vi "Byte Array.vi"(8 "Error In":errorcluster) -> (0 "Error Out":errorcluster)   [LabVIEW 2017, in "Tests.lvlib" / "To Msgpack.lvlib"]
uses:
  To Msgpack.lvlib
  <vilib>/addons/_JKI Toolkits/Caraya/classes/Test/Test.lvclass
  src/LabPack/LabPack.lvlib
  <vilib>/addons/_JKI Toolkits/Caraya/classes/Assert/Assert.lvclass
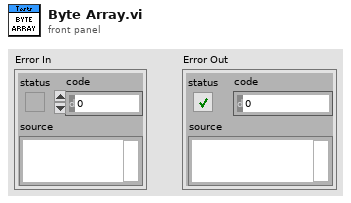
[diagram p1: front panel]
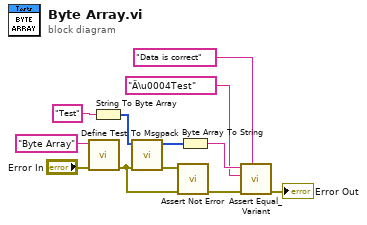
[diagram p0: block diagram]
diagram:
  n1 = call <vilib>:"Define Test.vi"("error in (no error)"="Error In", "Label (VI Title)"="Byte Array") -> ("error out"=w8:errorcluster)  [unwired: 9 in]
  n2 = String To Byte Array(string="Test") -> (unsigned byte array=w1:u8[])
  n3 = call "To Msgpack.vi"("Error In"=w8, "Anything"=w1) -> ("Error Out"=w9:errorcluster, "Msgpack Data"=w6:u8[])  [unwired: 8 in]
  n4 = call <vilib>:"Assert Not Error.vi"("error in (no error)"=w8, "Not Error?"=w9) -> ("error out"=w10:errorcluster)  [unwired: 9 in]
  n5 = Byte Array To String(unsigned byte array=w6) -> (string=w5:string)
  n6 = call <vilib>:"Assert Equal_Variant.vi"("Label"="Data is correct", "error in (no error)"=w10, "Y"="Ä\u0004Test" ("string"), "X"=w5) -> ("error out"=→"Error Out":errorcluster)  [unwired: 7 in]
